vi "AppendToHDF5.vi"(7 "det_hardware":enum16{"CAMERA", "PMT"}(ring), 8 "error in (no error)":errorcluster, 9 "PMT IN":i16[][](array[numeric]), 10 "Camera in":i16[][][][](array[numeric]), 11 "appended path":path) -> (0 "error out":errorcluster)   [LabVIEW 2019]
uses:
  <vilib>/UPVI/lvhdf5/file.llb/LVH5F Operation.ctl
  <vilib>/UPVI/lvhdf5/dataset.llb/Append Element(s) to Dataset (Variant).vi
  <vilib>/UPVI/lvhdf5/dataset.llb/Append Element(s) to Dataset.xnode
  <vilib>/UPVI/lvhdf5/library.llb/HDF5 Ref.ctl
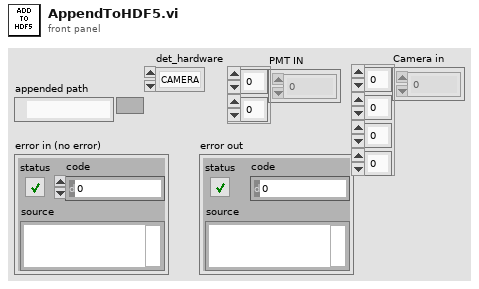
[diagram p1: front panel]
types:
  T1 = typedef "LVH5F Operation.ctl" = enum16{"open", "open or create", "create or replace", "create or replace (with confirmation)", "create", "open (read only)"}
  T2 = typedef "HDF5 Ref.ctl" = refnum<k1>
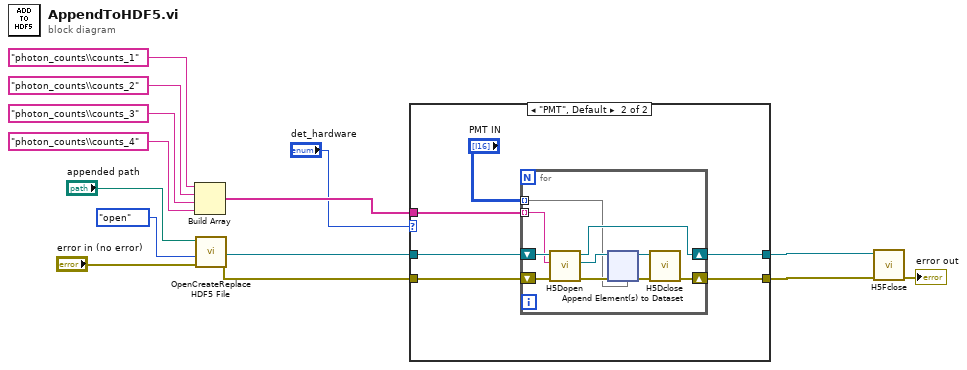
[diagram p0: block diagram]
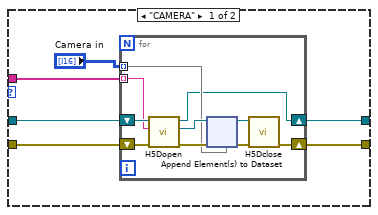
[diagram p2: hidden frame]
diagram:
  n1 = Build Array("photon_counts\\counts_1" ("Dataset Path"), "photon_counts\\counts_2" ("Dataset Path"), "photon_counts\\counts_3" ("Dataset Path"), "photon_counts\\counts_4" ("Dataset Path")) -> (w4:string[])
  n2 = call <vilib>:"OpenCreateReplace HDF5 File.vi"("error in (no error)"="error in (no error)", "function (open or create)"=LVH5F_Operation."open", "path"="appended path") -> ("error out"=w14:errorcluster, "HDF5 Ref out"=w13:T2)  [unwired: 5 in]
  n3 = case shown="\"PMT\", Default" "det_hardware" {
    tunnel: w14 -> [w20 w44]
    tunnel: w13 -> [w19 w43]
    tunnel: w4 -> [w18 w42]
    tunnel: [w16 w41] -> w3
    tunnel: [w15 w40] -> w2
    frame "CAMERA" {
      n4 = for {
        tunnel: w18 -> [w26] mode=indexing
        tunnel: "Camera in" -> [w25] mode=indexing
        shift-right: [w23] -> w15
        shift-left: w20 -> [w28]
        shift-right: [w21] -> w16
        shift-left: w19 -> [w27]
        n5 = call <vilib>:"H5Dopen.vi"("error in (no error)"=w28, "name"=w26, "HDF5 Ref"=w27) -> ("error out"=w29:errorcluster, "HDF5 Dataset Ref"=w30:T2, "HDF5 Ref out"=w21:T2)  [unwired: 4 in]
        n6 = xnode "Append Element(s) to Dataset"("HDF5 Dataset Ref"=w30, "error in (no error)"=w29, "Data Element(s)"=w25) -> ("HDF5 Dataset out"=w22:T2, "error out"=w24:errorcluster)  [unwired: 1 in, 2 out]
        n7 = call <vilib>:"H5Dclose.vi"("error in (no error)"=w24, "HDF5 Dataset Ref"=w22) -> ("error out"=w23:errorcluster)  [unwired: 7 in]
      }
    }
    frame "PMT", Default {
      n8 = for {
        tunnel: w42 -> [w50] mode=indexing
        shift-right: [w48] -> w40
        shift-left: w44 -> [w52]
        shift-right: [w46] -> w41
        shift-left: w43 -> [w51]
        tunnel: "PMT IN" -> [w45] mode=indexing
        n9 = call <vilib>:"H5Dopen.vi"("error in (no error)"=w52, "name"=w50, "HDF5 Ref"=w51) -> ("error out"=w53:errorcluster, "HDF5 Dataset Ref"=w54:T2, "HDF5 Ref out"=w46:T2)  [unwired: 4 in]
        n10 = xnode "Append Element(s) to Dataset"("HDF5 Dataset Ref"=w54, "error in (no error)"=w53, "Data Element(s)"=w45) -> ("HDF5 Dataset out"=w47:T2, "error out"=w49:errorcluster)  [unwired: 1 in, 2 out]
        n11 = call <vilib>:"H5Dclose.vi"("error in (no error)"=w49, "HDF5 Dataset Ref"=w47) -> ("error out"=w48:errorcluster)  [unwired: 7 in]
      }
    }
  }
  n12 = call <vilib>:"H5Fclose.vi"("error in (no error)"=w2, "HDF5 Ref"=w3) -> ("error out"=→"error out":errorcluster)  [unwired: 7 in]
